vi "sort_2d_cell_details_array.vi"(9 "Column descending? array":bool[](array[boolean]), 10 "Column priority array":dbl[](array[numeric]), 11 "Unsorted Array":string[][](array[string])) -> (3 "Sorted Array":string[][](array[string]))   [LabVIEW 2016]
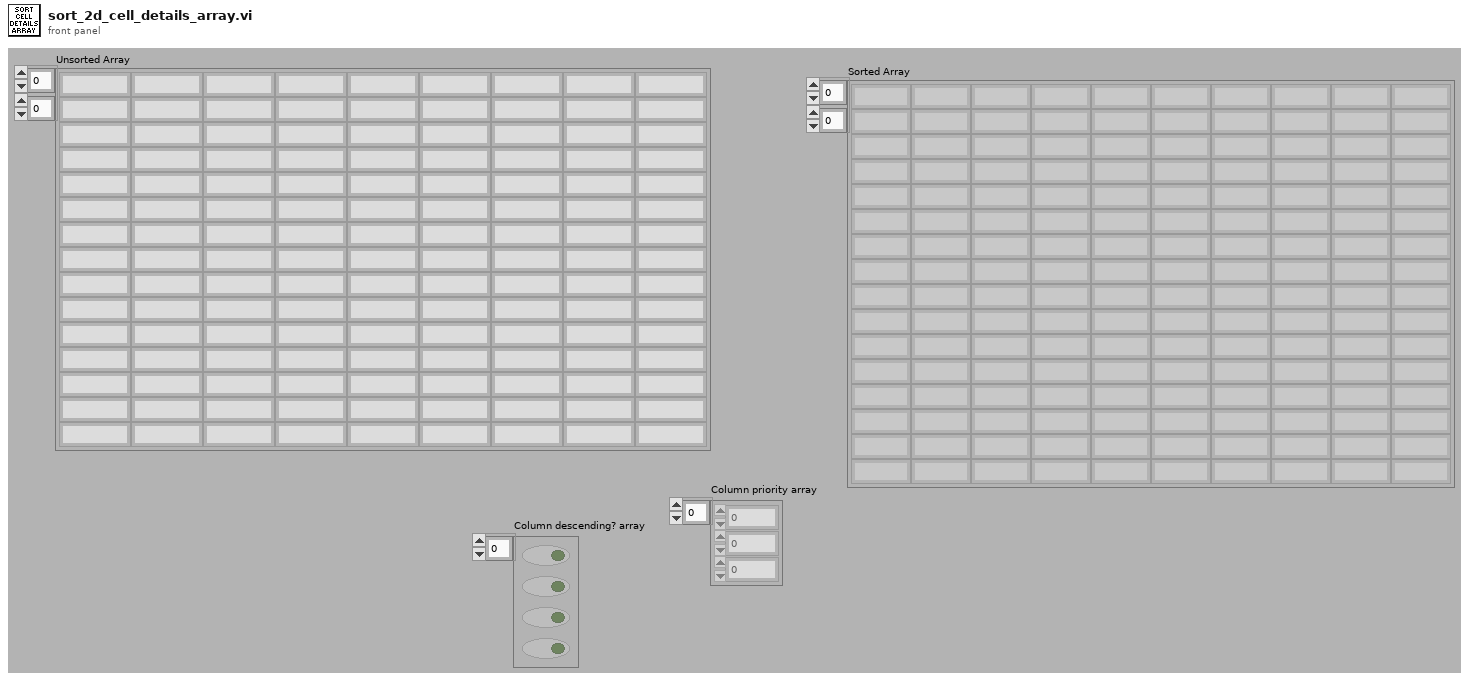
[diagram p1: front panel]
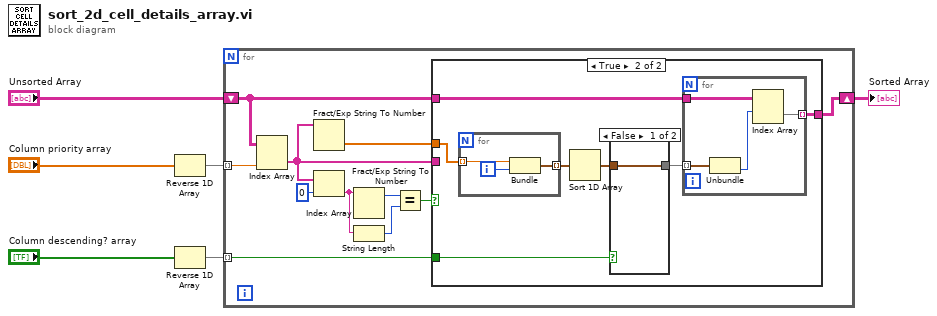
[diagram p0: block diagram]
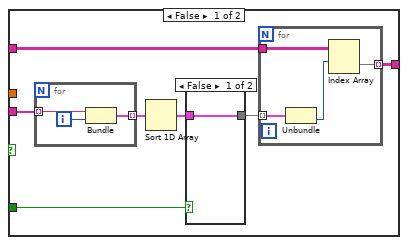
[diagram p2: hidden frame]
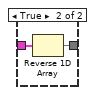
[diagram p3: hidden frame]
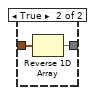
[diagram p4: hidden frame]
diagram:
  n1 = Reverse 1D Array(array="Column priority array") -> (reversed array=w6:dbl[])
  n2 = Reverse 1D Array(array="Column descending? array") -> (reversed array=w5:bool[])
  n3 = for {
    shift-right: [w15] -> w2
    shift-left: "Unsorted Array" -> [w17]
    tunnel: w6 -> [w16] mode=indexing
    tunnel: w5 -> [w14] mode=indexing
    n4 = Index Array(array=w17, index (col)=w16) -> (element=w12:string[])  [unwired: 1 in]
    n5 = Fract/Exp String To Number(string=w12) -> (number=w13:dbl[])  [unwired: 3 in, 1 out]
    n6 = Index Array(array=w12, index=0) -> (element=w10:string)
    n7 = Fract/Exp String To Number(string=w10) -> (offset past number=w9:i32)  [unwired: 3 in, 1 out]
    n8 = String Length(string=w10) -> (length=w8:i32)
    n9 = Equal?(x=w9, y=w8) -> (x = y?=w7:bool)
    n10 = case shown="True" w7 {
      tunnel: w17 -> [w23 w41]
      tunnel: [w22 w35] -> w15
      tunnel: w12 -> [w21 _]
      tunnel: w14 -> [w18 w36]
      tunnel: w13 -> [_ w40]
      frame False {
        n11 = for {
          tunnel: w21 -> [w33] mode=indexing
          tunnel: [w34] -> w24 mode=indexing
          i -> [w32]
          n12 = Bundle("String"=w33, w32) -> (w34:cluster{"String":string, i32})  [unwired: 1 out]
        }
        n13 = Sort 1D Array(array=w24) -> (sorted array=w20:cluster{"String":string, i32}[])
        n14 = case shown="False" w18 {
          tunnel: w20 -> [w25 w27]
          tunnel: [w25 w26] -> w19
          frame False {
          }
          frame True {
            n15 = Reverse 1D Array(array=w27) -> (reversed array=w26:cluster{"String":string, i32}[])
          }
        }
        n16 = for {
          tunnel: w19 -> [w31] mode=indexing
          tunnel: w23 -> [w30]
          tunnel: [w28] -> w22 mode=indexing
          n17 = Unbundle(w31) -> (w29:i32)  [unwired: 1 out]
          n18 = Index Array(array=w30, index (row)=w29) -> (element=w28:string[])  [unwired: 1 in]
        }
      }
      frame True {
        n19 = for {
          tunnel: w40 -> [w50] mode=indexing
          tunnel: [w51] -> w39 mode=indexing
          i -> [w49]
          n20 = Bundle("String"=w50, w49) -> (w51:cluster{"String":dbl, i32})  [unwired: 1 out]
        }
        n21 = Sort 1D Array(array=w39) -> (sorted array=w38:cluster{"String":dbl, i32}[])
        n22 = case shown="False" w36 {
          tunnel: w38 -> [w42 w44]
          tunnel: [w42 w43] -> w37
          frame False {
          }
          frame True {
            n23 = Reverse 1D Array(array=w44) -> (reversed array=w43:cluster{"String":dbl, i32}[])
          }
        }
        n24 = for {
          tunnel: w37 -> [w48] mode=indexing
          tunnel: w41 -> [w47]
          tunnel: [w45] -> w35 mode=indexing
          n25 = Unbundle(w48) -> (w46:i32)  [unwired: 1 out]
          n26 = Index Array(array=w47, index (row)=w46) -> (element=w45:string[])  [unwired: 1 in]
        }
      }
    }
  }
  "Sorted Array" <- w2
